vi "AderlingCapacitance.vi"(1 "GPIB Address":string) -> (0 "Numeric":dbl)   [LabVIEW 2015]
panel:
  out "Numeric 3":i32
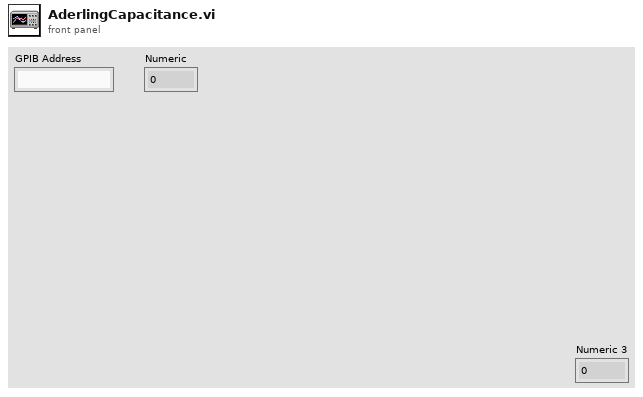
[diagram p1: front panel]
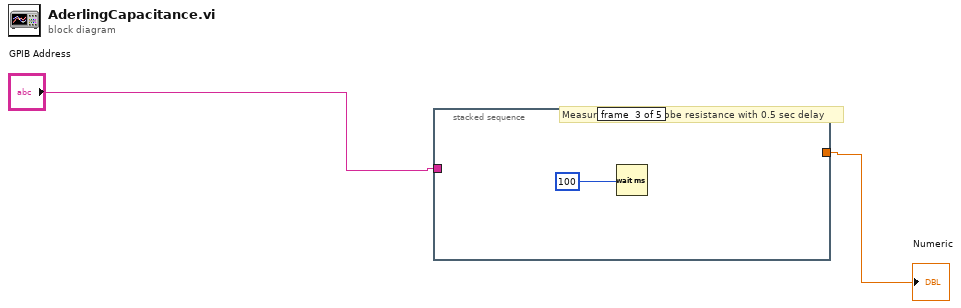
[diagram p0: block diagram]
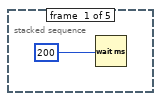
[diagram p2: hidden frame]
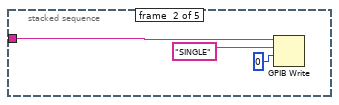
[diagram p3: hidden frame]
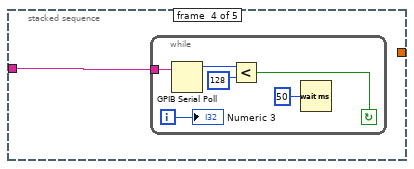
[diagram p4: hidden frame]
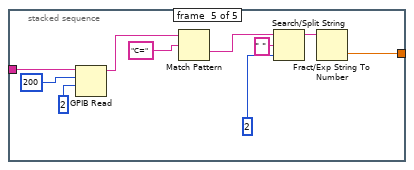
[diagram p5: hidden frame]
diagram:
  # "Measure Keithley 2probe resistance with 0.5 sec delay"
  n1 = stacked-sequence {
    tunnel: [_ _ _ _ w20] -> w2
    tunnel: "GPIB Address" -> [_ w4 _ w8 w16]
    frame #0 {
      n2 = Wait (ms)(milliseconds to wait=200) -> ()  [unwired: 1 out]
    }
    frame #1 {
      n3 = GPIB Write(0:w4, 1:"SINGLE" ("data"), 2:i16 0 ("mode (0)")) -> ()  [unwired: 2 in, 2 out]
    }
    frame #2 {
      n4 = Wait (ms)(milliseconds to wait=100) -> ()  [unwired: 1 out]
    }
    frame #3 {
      n5 = while {
        tunnel: w8 -> [w9]
        i -> [w10]
        stop <- w12 continue-if-true
        n6 = GPIB Serial Poll(0:w9) -> (2:w14:i16)  [unwired: 1 in, 2 out]
        n7 = Less?(x=w14, y=i16 128) -> (x < y?=w12:bool)
        n8 = Wait (ms)(milliseconds to wait=u32 50) -> ()  [unwired: 1 out]
        "Numeric 3" <- w10
      }
    }
    frame #4 {
      n9 = GPIB Read(0:w16, 1:200 ("byte count"), 2:i16 2 ("mode (0)")) -> (5:w19:string)  [unwired: 2 in, 2 out]
      n10 = Match Pattern(string=w19, regular expression="C=") -> (after substring=w18:string)  [unwired: 1 in, 3 out]
      n11 = Search/Split String(string=w18, search string/char (-)=" ", offset (0)=i16 2 ("mode (0)")) -> (substring before match=w21:string)  [unwired: 2 out]
      n12 = Fract/Exp String To Number(string=w21) -> (number=w20:dbl)  [unwired: 3 in, 1 out]
    }
  }
  "Numeric" <- w2
